vi "PlLoN_grabber_recoveryTRYFIX.vi"(7 "Number of Images":u32=1 min=1 step=1, 8 "error in (no error)":errorcluster, 10 "refnum":refnum<file>, 11 "Camera Handle":u32) -> (0 "error out":errorcluster, 1 "DATA":u16[][](array[numeric]), 2 "Number of Images":u32=1 min=1 step=1, 3 "Camera Handle":u32, 4 "x/y":dbl, 5 "refnum out":refnum<file>, 6 "x > y?":bool)   [LabVIEW 2015]
panel:
  out "Waveform Graph":dbl[][](graph)
  out "PyLoN Ready":bool
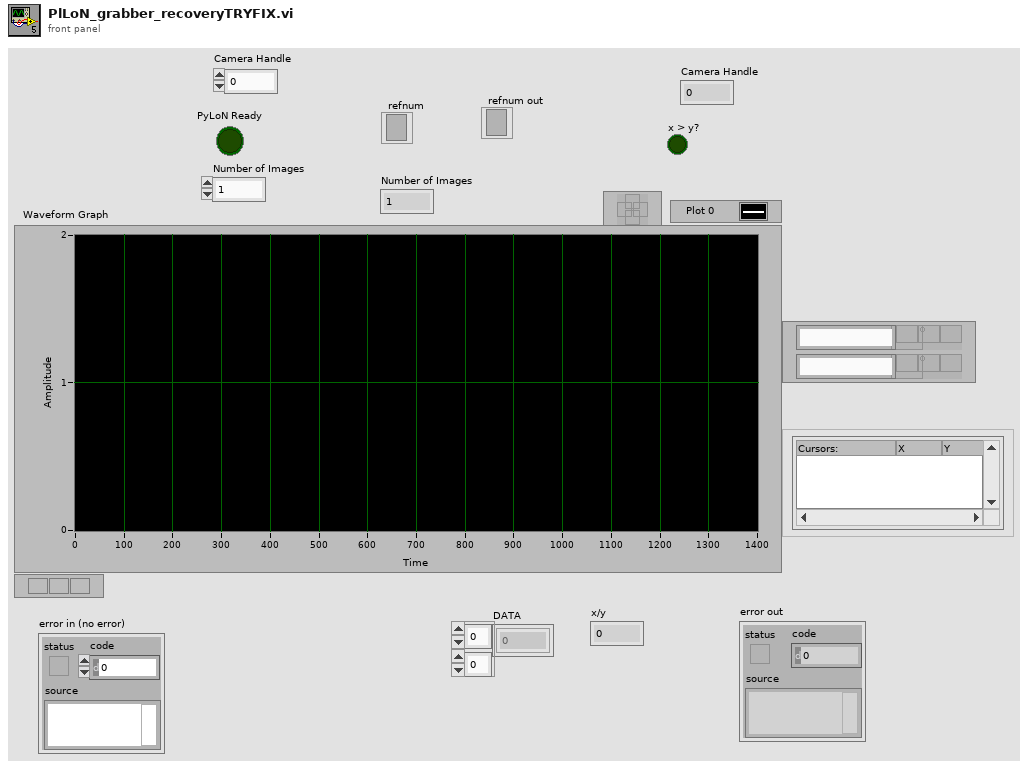
[diagram p1: front panel]
types:
  T1 = cluster{"acquire focus mode":u32, "Exposure Time (s)":dbl, "Number of Images":u32, "Software accumulation":u32}
  T2 = cluster{"Camera Handle":u32, "Pulser Handle":u32, "File Handle":u32, "Display Handle":u32, "Image Handle":u32}
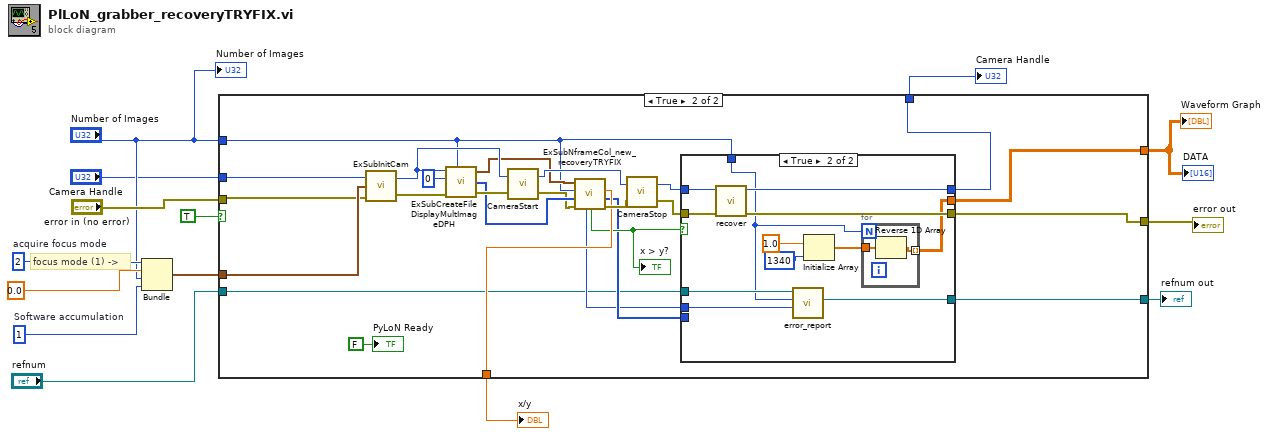
[diagram p0: block diagram]
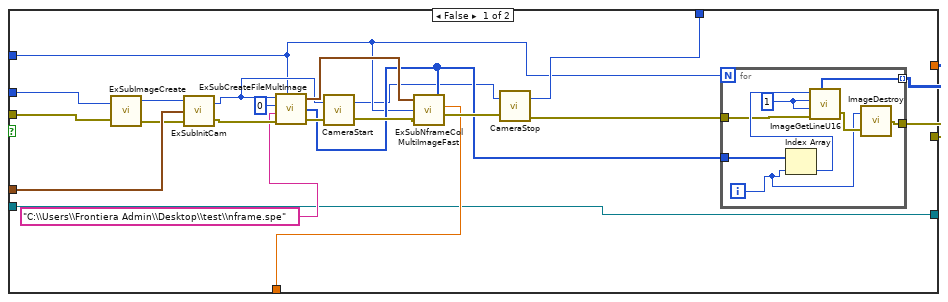
[diagram p2: hidden frame]
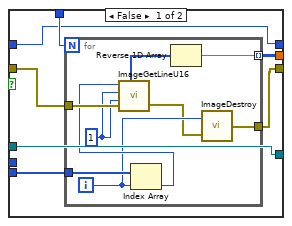
[diagram p3: hidden frame]
diagram:
  w8 = u32 2  # acquire focus mode
  w9 = u32 1  # Software accumulation
  # "focus mode (1) ->"
  n1 = Bundle("acquire focus mode"=w8, "Exposure Time (s)"=0.0, "Number of Images"="Number of Images", "Software accumulation"=w9) -> (w7:T1)  [unwired: 1 in]
  n2 = case shown="True" TRUE {
    tunnel: [w21 w47] -> w3
    tunnel: [w19 w51] -> w14
    tunnel: [w20 w50] -> w13
    tunnel: "Number of Images" -> [w17 w49]
    tunnel: [w18 w58] -> w12
    tunnel: "error in (no error)" -> [w36 w56]
    tunnel: w7 -> [w34 w63]
    tunnel: "Camera Handle" -> [w32 w57]
    tunnel: "refnum" -> [w15 w45]
    tunnel: [w15 w46] -> w1
    frame False {
      n3 = call "ExSubImageCreate.vi"("Camera Handle"=w32, "error in (no error)"=w36) -> ("Camera Handle"=w35:u32, "error out"=w33:errorcluster)  [unwired: 1 out]
      n4 = call "ExSubInitCam.vi"("error in (no error)"=w33, "Camera Information"=w34, "Camera Handle"=w35) -> ("error out"=w31:errorcluster, "Camera Handle"=w25:u32)
      n5 = call "ExSubCreateFileMultImage.vi"("Camera Handle"=w25, "Pulser Handle"=u32 0, "File and Display Name"="C:\\Users\\Frontiera Admin\\Desktop\\test\\nframe.spe", "error in (no error)"=w31, "Number of Images"=w17) -> ("Handles Out"=w26:T2, "Array"=w23:u32[], "error out"=w28:errorcluster)
      n6 = call <userlib>:"CameraStart.vi"("error in"=w28, "Camera Handle"=w25) -> ("error out"=w27:errorcluster, "Camera Handle"=w16:u32)
      n7 = call "ExSubNframeColMultiImageFast.vi"("Handle Cluster"=w26, "Number of Images"=w17, "error in (no error)"=w27, "image handles"=w23) -> ("x/y"=w18:dbl, "error out"=w24:errorcluster)  [unwired: 1 out]
      n8 = call <userlib>:"CameraStop.vi"("error in"=w24, "Camera Handle"=w16) -> ("error out"=w22:errorcluster, "Camera Handle"=w19:u32)
      n9 = for {
        N: w17 -> [_]
        tunnel: w23 -> [w44]
        tunnel: w22 -> [w41]
        tunnel: [w40] -> w21 mode=indexing
        tunnel: [w38] -> w20
        i -> [w37]
        w42 = u32 1 ("Y Position")
        n10 = Index Array(array=w44, index=w37) -> (element=w43:u32)
        n11 = call <userlib>:"ImageGetLineU16.vi"("Data Handle"=w43, "Y Position"=w42, "Z Position"=w42, "error in"=w41) -> ("Array u16"=w40:u16[], "error out"=w39:errorcluster)  [unwired: 1 out]
        n12 = call <userlib>:"ImageDestroy.vi"("error in"=w39, "Data handle"=w37) -> ("error out"=w38:errorcluster)
      }
    }
    frame True {
      n13 = call "ExSubInitCam.vi"("error in (no error)"=w56, "Camera Information"=w63, "Camera Handle"=w57) -> ("error out"=w67:errorcluster, "Camera Handle"=w65:u32)
      n14 = call "ExSubCreateFileDisplayMultImageDPH.vi"("Camera Handle"=w65, "Pulser Handle"=u32 0, "error in (no error)"=w67, "Number of Images"=w49) -> ("Handles Out"=w62:T2, "Array"=w61:u32[], "error out"=w66:errorcluster)  [unwired: 1 in]
      n15 = call <userlib>:"CameraStart.vi"("error in"=w66, "Camera Handle"=w65) -> ("error out"=w60:errorcluster, "Camera Handle"=w68:u32)
      n16 = call "ExSubNframeCol_new_recoveryTRYFIX.vi"("error in (no error)"=w60, "image handles"=w61, "Number of Images"=w49, "Handle Cluster 2"=w62) -> ("error out"=w59:errorcluster, "data handles"=w52:u32[], "x/y"=w58:dbl, "x > y?"=w54:bool, "image #"=w48:i32)  [unwired: 2 in, 1 out]
      "x > y?" <- w54
      n17 = call <userlib>:"CameraStop.vi"("error in"=w59, "Camera Handle"=w68) -> ("error out"=w55:errorcluster, "Camera Handle"=w53:u32)
      n18 = case shown="True" w54 {
        tunnel: w55 -> [w75 w95]
        tunnel: [w74 w94] -> w50
        tunnel: w53 -> [w71 w97]
        tunnel: [w71 w96] -> w51
        tunnel: w52 -> [w76 _]
        tunnel: w49 -> [w73 w89]
        tunnel: w48 -> [_ w86]
        tunnel: w45 -> [w70 w91]
        tunnel: [w72 w87] -> w47
        tunnel: [w70 w90] -> w46
        frame False {
          n19 = for {
            N: w73 -> [_]
            tunnel: w76 -> [w82]
            tunnel: w75 -> [w85]
            tunnel: [w77] -> w72 mode=indexing
            tunnel: [w79] -> w74
            i -> [w81]
            w84 = u32 1
            n20 = Index Array(array=w82, index=w81) -> (element=w83:u32)
            n21 = call <userlib>:"ImageGetLineU16.vi"("Data Handle"=w83, "Y Position"=w84, "Z Position"=w84, "error in"=w85) -> ("Array u16"=w78:u16[], "error out"=w80:errorcluster)  [unwired: 1 out]
            n22 = Reverse 1D Array(array=w78) -> (reversed array=w77:u16[])
            n23 = call <userlib>:"ImageDestroy.vi"("error in"=w80, "Data handle"=w81) -> ("error out"=w79:errorcluster)
          }
        }
        frame True {
          n24 = call "recover.vi"("error in (no error)"=w95, "Camera Handle"=w97) -> ("error out"=w94:errorcluster, "Camera Handle"=w96:u32)  [unwired: 7 in, 1 out]
          n25 = call "error_report.vi"("frame #"=w86, "# of frame"=w89, "refnum"=w91) -> ("refnum out"=w90:refnum<file>)  [unwired: 7 in, 1 out]
          n26 = Initialize Array(1.0 ("element"), 1340 ("dimension size")) -> (w88:dbl[])
          n27 = for {
            N: w89 -> [_]
            tunnel: w88 -> [w98]
            tunnel: [w99] -> w87 mode=indexing
            n28 = Reverse 1D Array(array=w98) -> (reversed array=w99:dbl[])
          }
        }
      }
      "PyLoN Ready" <- FALSE ("PyLoN Ready")
    }
  }
  "error out" <- w13
  "DATA" <- w3
  "Camera Handle" <- w14
  "x/y" <- w12
  "Waveform Graph" <- w3
  "refnum out" <- w1
  "Number of Images" <- "Number of Images"
